vi "Fetch Multiple Points.vi"(8 "error in (no error)":errorcluster, 9 "Timeout (20000 ms)":u32=20000, 11 "VISA resource name":refnum<visa-resource-name>) -> (0 "error out":errorcluster, 2 "Measurements":dbl[](array[numeric]), 3 "VISA resource name out":refnum<visa-resource-name>)   [LabVIEW 2021, in "Agilent 34420.lvlib"]
doc: "This low-level VI returns an array of values from a previously initiated measurement. The number of measurements the instrument takes is determined by the values you specify for the <B>Trigger Count</B> control and <B>Sample Count</B> control of the <B>Configure Multipoint</B> VI.\n\n<B>Note:</B>\n\nUse this VI only with other low-level VIs. The high-level VIs automatically incorporate this functionality. This VI does not check the instrument status. If you want to check the instrument status, call the Error Query VI at the conclusion of the sequence.\n\nIt is only possible to fetch a maximum of 1024 measurements from the internal buffer of the instrument. If you are using low level VIs such as <B>Initiate</B> and </B>Fetch Multiple Points</B>, you will get an error if the product of <B>Trigger Count</B> and <B>Sample Count</B> is greater than 1024. <B>Read</B> VI doesn't have a limit since it reads as measurements are being made."
uses:
  <instrlib>/Agilent 34420/Agilent 34420.lvlib
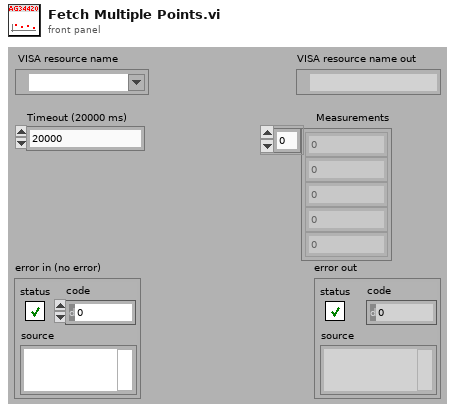
[diagram p1: front panel]
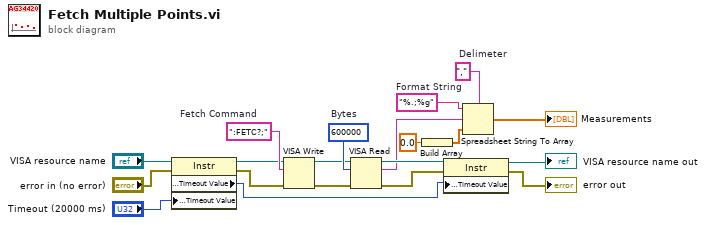
[diagram p0: block diagram]
diagram:
  w7 = ":FETC?;"  # Fetch Command
  w19 = ","  # Delimeter
  w20 = "%.;%g"  # Format String
  w8 = u32 600000  # Bytes
  n1 = property class="Instr"(reference="VISA resource name", error in="error in (no error)", "General Settings:Timeout Value"="Timeout (20000 ms)") -> (reference out=w4:refnum<visa-resource-name>, error out=w3:errorcluster, "General Settings:Timeout Value"=w12:u32)
  n2 = VISA Write(VISA resource name=w4, write buffer=w7, error in (no error)=w3) -> (VISA resource name out=w2:refnum<visa-resource-name>, error out=w1:errorcluster)  [unwired: 1 out]
  n3 = VISA Read(VISA resource name=w2, byte count=w8, error in (no error)=w1) -> (VISA resource name out=w14:refnum<visa-resource-name>, read buffer=w9:string, error out=w13:errorcluster)  [unwired: 1 out]
  n4 = Build Array(0.0) -> (w17:dbl[])
  n5 = property class="Instr"(reference=w14, error in=w13, "General Settings:Timeout Value"=w12) -> (reference out=→"VISA resource name out":refnum<visa-resource-name>, error out=→"error out":errorcluster)
  n6 = Spreadsheet String To Array(delimiter (Tab)=w19, format string=w20, spreadsheet string=w9, array type (2D Dbl)=w17) -> (array=→"Measurements":dbl[])
